vi "Array of Variants to Cluster Variant.vi"(8 "error in (no error)":errorcluster, 11 "[Variant]":variant[](array[variant])) -> (0 "error out":errorcluster, 3 "Cluster Variant":variant)   [LabVIEW 2018, in "TwinCAT ADS.lvclass"]
uses:
  TwinCAT ADS.lvclass
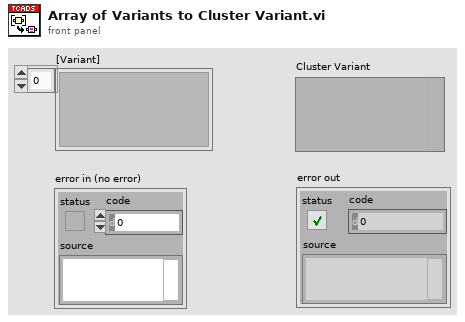
[diagram p1: front panel]
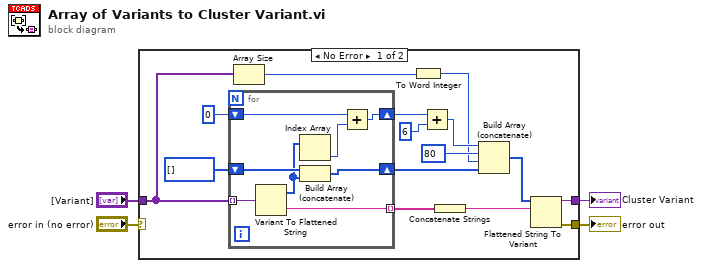
[diagram p0: block diagram]
diagram:
  n1 = case shown="No Error" "error in (no error)" {
    selector: "error in (no error)" -> [_ w28]
    tunnel: [w14 w28] -> w4
    tunnel: [w15 _] -> w3
    tunnel: "[Variant]" -> [w13 _]
    frame No Error {
      n2 = for {
        tunnel: w13 -> [w27] mode=indexing
        shift-right: [w22] -> w17
        shift-left: i16 0 -> [w23]
        shift-right: [w21] -> w11
        shift-left: i16[] [] ("type string") -> [w26]
        tunnel: [w20] -> w6 mode=indexing
        n3 = Variant To Flattened String(Variant=w27) -> (data string=w20:string, 1:w25:i16[])
        n4 = Index Array(array=w25) -> (element=w24:i16)  [unwired: 1 in]
        n5 = Build Array (concatenate)(w26, w25) -> (w21:i16[])
        n6 = Add(x=w23, y=w24) -> (x+y=w22:i16)
      }
      n7 = Array Size(array=w13) -> (size(s)=w12:i32)
      n8 = To Word Integer(number=w12) -> (16bit integer=w7:i16)
      n9 = Add(x=w17, y=i16 6) -> (x+y=w9:i16)
      n10 = Concatenate Strings(w6) -> (w5:string)
      n11 = Build Array (concatenate)(w9, i16 80, w7, w11) -> (w10:i16[])
      n12 = Flattened String To Variant(6:w5, 7:w10) -> (0:w14:errorcluster, 3:w15:variant)  [unwired: 1 in]
    }
    frame Error {
    }
  }
  "Cluster Variant" <- w3
  "error out" <- w4
